vi "ShowManual.vi"(8 "error in (no error)":errorcluster caption="错误输入（无错误）", 9 "坐标":T1, 10 "菜单引用":refnum<k9>, 11 "DigitalDisplay 输入":refnum<class "DigitalDisplay.lvclass">) -> (0 "error out":errorcluster caption="错误输出", 3 "DigitalDisplay 输出":refnum<class "DigitalDisplay.lvclass">)   [LabVIEW 2018, in "DataDisplay.lvlib" / "DigitalDisplay.lvclass"]
uses:
  DigitalDisplay.lvclass
  <vilib>/Utility/miscctls.llb/LVPoint32TypeDef.ctl
  DigitalDisplay.lvclass/DigitalDisplay.ctl
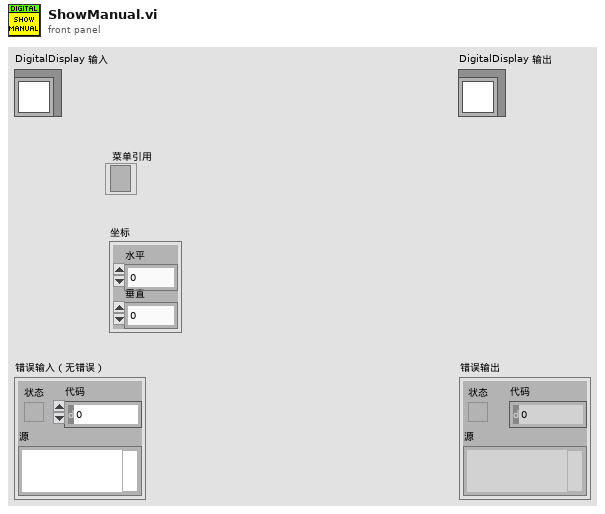
[diagram p1: front panel]
types:
  T1 = typedef "LVPoint32TypeDef.ctl" = cluster{"Horizontal":i32, "Vertical":i32}
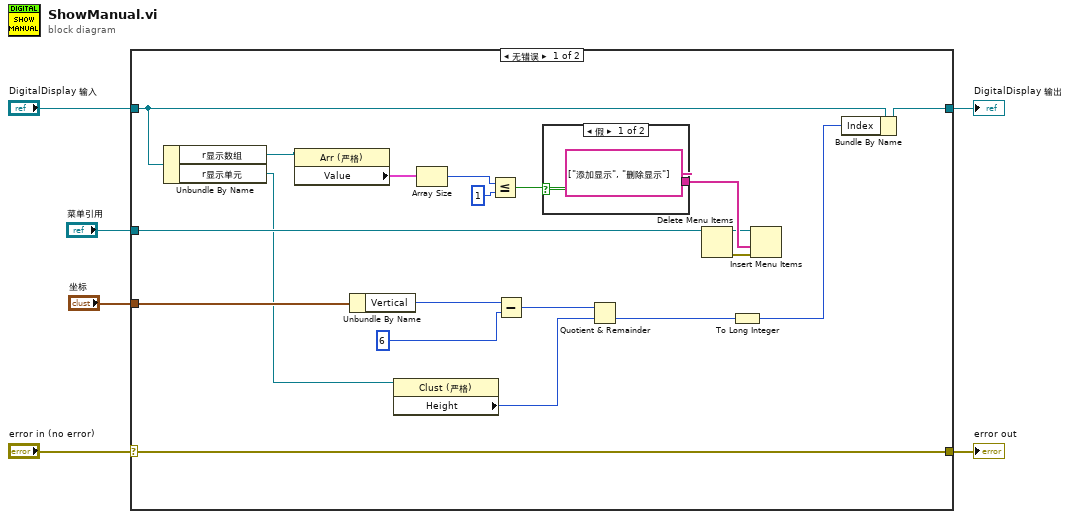
[diagram p0: block diagram]
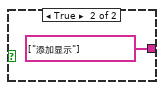
[diagram p2: hidden frame]
diagram:
  n1 = case shown="无错误" "error in (no error)" {
    selector: "error in (no error)" -> [w26 w30]
    tunnel: [w26 w30] -> w5
    tunnel: [w9 w29] -> w3
    tunnel: "DigitalDisplay 输入" -> [w12 w29]
    tunnel: "坐标" -> [w14 _]
    tunnel: "菜单引用" -> [w13 _]
    frame No Error {
      n2 = Unbundle By Name(w12) -> ("r显示数组"=w11:refnum<vi>, "r显示单元"=w10:refnum<vi>)
      n3 = property class="Arr (严格)"(reference=w11) -> ("Value"=w25:cluster{"通道选择":u16, "数值":string}[])  [unwired: 1 in, 2 out]
      n4 = Unbundle By Name(w14) -> ("Vertical"=w18:i32)
      n5 = property on="属性节点" class="Clust (严格)"(reference=w10) -> ("Height"=w15:u32)  [unwired: 1 in, 2 out]
      n6 = Array Size(array=w25) -> (size(s)=w24:i32)
      n7 = Less Or Equal?(x=w24, y=1) -> (x <= y?=w22:bool)
      n8 = Subtract(x=w18, y=6) -> (x-y=w17:i32)
      n9 = case shown="假" w22 {
        tunnel: [string[] ["添加显示", "删除显示"] ("项标识符") string[] ["添加显示"] ("项标识符")] -> w21
        frame False {
        }
        frame True {
        }
      }
      n10 = Quotient & Remainder(x=w17, y=w15) -> (floor(x/y)=w8:u32)  [unwired: 1 out]
      n11 = Delete Menu Items(9:w13) -> (0:w19:errorcluster, 3:w20:refnum<k9>)  [unwired: 3 in]
      n12 = To Long Integer(number=w8) -> (32bit integer=w7:i32)
      n13 = Insert Menu Items(6:w19, 7:w21, 9:w20) -> ()  [unwired: 3 in, 3 out]
      n14 = Bundle By Name(cluster=w12, "Index"=w7) -> (w9:refnum<class "DigitalDisplay.lvclass">)
    }
    frame Error {
    }
  }
  "error out" <- w5
  "DigitalDisplay 输出" <- w3
